vi "ISX3_Connect.vi"(3 "Connect to device with\nFT_Handle":u32) -> (1 "Connected to device:":u32)   [LabVIEW 2012, in "Sciospec ISX3 Impedance Analyzer.lvlib"]
uses:
  Sciospec ISX3 Impedance Analyzer.lvlib
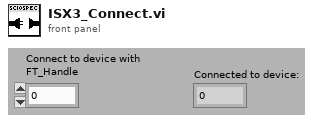
[diagram p1: front panel]
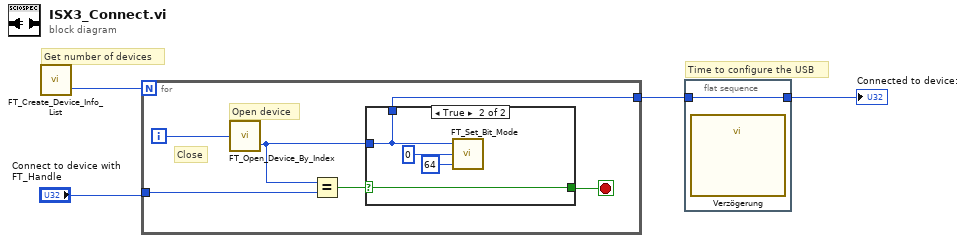
[diagram p0: block diagram]
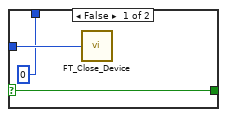
[diagram p2: hidden frame]
diagram:
  # "Time to configure the USB"
  # "Get number of devices"
  n1 = call "FT_Create_Device_Info_List.vi"() -> ("Number of Devices"=w4:u32)  [unwired: 1 out]
  n2 = for {
    N: w4 -> [_]
    tunnel: "Connect to device with\nFT_Handle" -> [w9]
    tunnel: [w5] -> w2
    i -> [w10]
    stop <- w7 stop-if-true
    # "Close"
    # "Open device"
    n3 = call "FT_Open_Device_By_Index.vi"("Device Index"=w10) -> ("Handle"=w6:u32)  [unwired: 1 out]
    n4 = Equal?(x=w6, y=w9) -> (x = y?=w8:bool)
    n5 = case shown="True" w8 {
      selector: w8 -> [w13 w17]
      tunnel: w6 -> [w12 w14]
      tunnel: [w13 w17] -> w7
      tunnel: [u32 0 w14] -> w5
      frame False {
        n6 = call "FT_Close_Device.vi"("Handle"=w12) -> ()  [unwired: 1 out]
      }
      frame True {
        n7 = call "FT_Set_Bit_Mode.vi"("Bit Mode"=u8 64 ("Enable"), "Bit Mode Mask"=u8 0 ("Mask"), "Handle"=w14) -> ()  [unwired: 1 out]
      }
    }
  }
  n8 = flat-sequence {
    tunnel: [w18] -> w1
    tunnel: w2 -> [w18]
    frame #0 {
      n9 = call "Verzögerung"() -> ()  [unwired: 11 in, 1 out]
    }
  }
  "Connected to device:" <- w1
